vi "Get Value.vi"(5 "timeout":dbl[unit]=1.0, 7 "PV name":string, 8 "error in":errorcluster, 11 "Client in":refnum<class "Client.lvclass">) -> (0 "error out":errorcluster, 1 "timed out?":bool, 2 "Value out":refnum<class "Value.lvclass">, 3 "Client out":refnum<class "Client.lvclass">)   [LabVIEW 2020, in "Client.lvlib" / "Client.lvclass"]
uses:
  Client.lvclass
  Client.lvclass/Client.ctl
  Value/Value/Value.lvclass
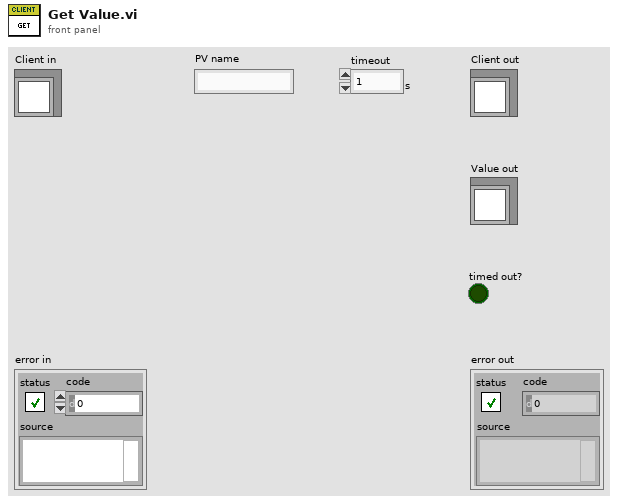
[diagram p1: front panel]
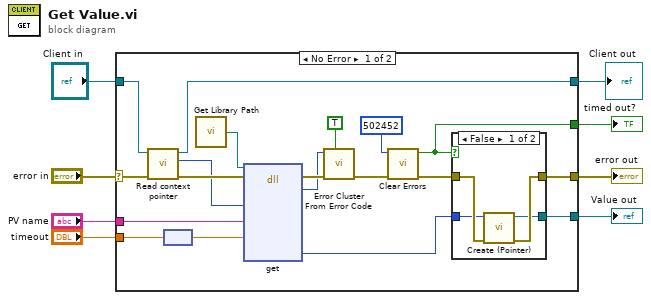
[diagram p0: block diagram]
diagram:
  n1 = case shown="No Error" "error in" {
    selector: "error in" -> [w27 w34]
    tunnel: [w11 w34] -> w5
    tunnel: [w22 w33] -> w4
    tunnel: "Client in" -> [w23 w33]
    tunnel: "PV name" -> [w24 _]
    tunnel: "timeout" -> [w19 _]
    tunnel: [w10 _] -> w2
    tunnel: [w9 _] -> w1
    frame No Error {
      n2 = call "Read context pointer.vi"("error in (no error)"=w27, "Client in"=w23) -> ("error out"=w26:errorcluster, "client pointer"=w25:i64, "Client out"=w22:refnum<class "Client.lvclass">)  [unwired: 7 in]
      n3 = node(w19) -> (w20:dbl)
      n4 = call "Get Library Path.vi"() -> ("Path"=w21:path)  [unwired: 1 in]
      n5 = dll-call lib="?" fn="get"(path in=w21, error in=w26, "client"=w25, "pv_name"=w24, "timeout"=w20) -> (error out=w17:errorcluster, "ret_code"=w16:i32, "value"=w15:i64)  [unwired: 5 in, 1 out]
      n6 = call <vilib>:"Error Cluster From Error Code.vi"("show call chain? (False)"=TRUE, "error in (no error)"=w17, "error code (0)"=w16) -> ("error out"=w14:errorcluster)  [unwired: 6 in]
      n7 = call <vilib>:"Clear Errors.vi"("error in (no error)"=w14, "specific error code to clear (0: all)"=502452) -> ("error out"=w12:errorcluster, "specific error cleared?"=w9:bool)  [unwired: 4 in]
      n8 = case shown="False" w9 {
        tunnel: w15 -> [w28 _]
        tunnel: w12 -> [w31 w32]
        tunnel: [w30 w32] -> w11
        tunnel: [w29 _] -> w10
        frame False {
          n9 = call "Create (Pointer).vi"("error in"=w31, "pointer"=w28) -> ("error out"=w30:errorcluster, "Value out"=w29:refnum<class "Value.lvclass">)  [unwired: 8 in]
        }
        frame True {
        }
      }
    }
    frame Error {
    }
  }
  "error out" <- w5
  "Client out" <- w4
  "Value out" <- w2
  "timed out?" <- w1
